vi "FT_Get_COM_Port_Number.vi"(0 "Handle":u32, 11 "Error In":errorcluster) -> (4 "FT_Status":u32(ring) items=["FT_OK", "FT_INVALID_HANDLE", "FT_DEVICE_NOT_FOUND", "FT_DEVICE_NOT_OPENED", "FT_IO_ERROR", "FT_INSUFFICIENT_RESOURCES", "FT_INVALID_PARAMETER", "FT_INVALID_BAUD_RATE", "FT_DEVICE_NOT_OPENED_FOR_ERASE", "FT_DEVICE_NOT_OPENED_FOR_WRITE", "FT_FAILED_TO_WRITE_DEVICE", "FT_EEPROM_READ_FAILED", "FT_EEPROM_WRITE_FAILED", "FT_EEPROM_ERASE_FAILED", "FT_EEPROM_NOT_PRESENT", "FT_EEPROM_NOT_PROGRAMMED", "FT_INVALID_ARGS", "FT_NOT_SUPPORTED", "FT_OTHER_ERROR"], 6 "COM Port Number":i32, 8 "COM Port String":string, 15 "Error Out":errorcluster)   [LabVIEW 2023, in "GEA2_Toolkit.lvlib"]
uses:
  library/GEA2_Toolkit.lvlib
  GEA3 DLL Source/ftd2xx.dll
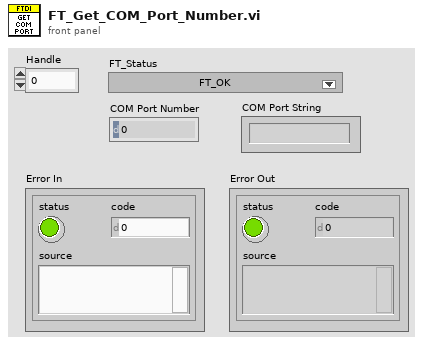
[diagram p1: front panel]
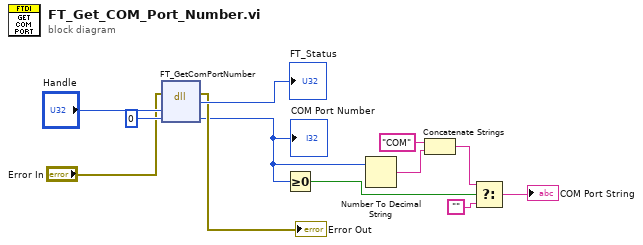
[diagram p0: block diagram]
diagram:
  n1 = dll-call lib="C:/TechnologyLab/NI-2010/Drivers/GEA3 Toolkit/GEA3 DLL Source/ftd2xx.dll" fn="FT_GetComPortNumber"(error in="Error In", "Handle"="Handle", "COM Port Number"=0) -> (error out=→"Error Out":errorcluster, "FT_Status"=→"FT_Status":u32, "COM Port Number"=w7:i32)  [unwired: 3 in, 1 out]
  "COM Port Number" <- w7
  n2 = Greater Or Equal To 0?(x=w7) -> (x >= 0?=w6:bool)
  n3 = Number To Decimal String(number=w7) -> (decimal integer string=w2:string)  [unwired: 1 in]
  n4 = Concatenate Strings("COM" ("string"), w2) -> (w1:string)
  n5 = Select(t=w1, s=w6, f="") -> (s? t:f=→"COM Port String":string)
